vi "Round_Min_Max.vi"(8 "Binning 1":u32(ring)=4 items=["1"=1, "2"=2, "4"=4, "10"=10], 10 "CrsList":T1, 11 "Use Cursors":bool) -> (0 "min(Y)":u32, 1 "max(Y)":u32, 2 "min(X)":u32, 3 "max(X)":u32)   [LabVIEW 2013]
uses:
  <vilib>/Utility/miscctls.llb/LVCursorListTypeDef.ctl
panel:
  # "Binning"
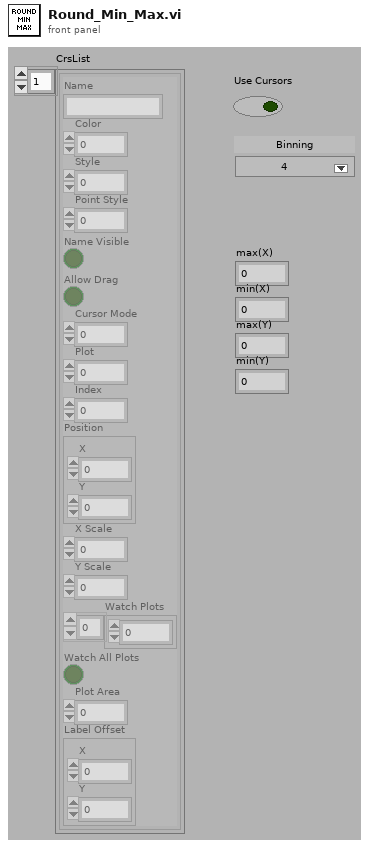
[diagram p1: front panel]
types:
  T1 = typedef "LVCursorListTypeDef.ctl" = cluster{"Name":string, "Color":u32, "Style":u8, "Point Style":u8, "Name Visible":bool, "Allow Drag":bool, "Cursor Mode":u32, "Plot":i32, "Index":i32, "Position":cluster{"X":dbl, "Y":dbl}, "X Scale":u32, "Y Scale":u32, "Watch Plots":i32[], "Watch All Plots":bool, "Plot Area":i32, "Label Offset":cluster{"X":dbl, "Y":dbl}}[]
  T2 = cluster{"Name":string, "Color":u32, "Style":u8, "Point Style":u8, "Name Visible":bool, "Allow Drag":bool, "Cursor Mode":u32, "Plot":i32, "Index":i32, "Position":cluster{"X":dbl, "Y":dbl}, "X Scale":u32, "Y Scale":u32, "Watch Plots":i32[], "Watch All Plots":bool, "Plot Area":i32, "Label Offset":cluster{"X":dbl, "Y":dbl}}
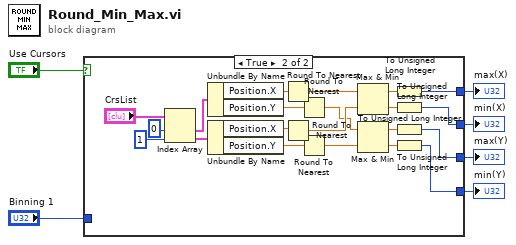
[diagram p0: block diagram]
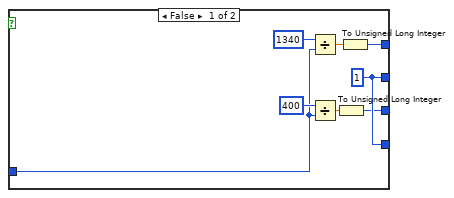
[diagram p2: hidden frame]
diagram:
  n1 = case shown="True" "Use Cursors" {
    tunnel: [w7 w18] -> w6
    tunnel: [w14 w15] -> w5
    tunnel: [w9 w16] -> w4
    tunnel: [w14 w17] -> w3
    tunnel: "Binning 1" -> [w11 _]
    frame False {
      w14 = u32 1
      n2 = Divide(x=u32 1340, y=w11) -> (x/y=w8:dbl)
      n3 = Divide(x=u32 400, y=w11) -> (x/y=w10:dbl)
      n4 = To Unsigned Long Integer(number=w10) -> (unsigned 32bit integer=w9:u32)
      n5 = To Unsigned Long Integer(number=w8) -> (unsigned 32bit integer=w7:u32)
    }
    frame True {
      n6 = Index Array(array="CrsList", index #1=0 ("index"), index #2=1 ("index")) -> (element #1=w21:T2, element #2=w22:T2)
      n7 = Unbundle By Name(w21) -> ("Position.X"=w23:dbl, "Position.Y"=w24:dbl)
      n8 = Unbundle By Name(w22) -> ("Position.X"=w25:dbl, "Position.Y"=w26:dbl)
      n9 = Round To Nearest(number=w23) -> (nearest integer value=w32:dbl)
      n10 = Round To Nearest(number=w25) -> (nearest integer value=w34:dbl)
      n11 = Round To Nearest(number=w24) -> (nearest integer value=w33:dbl)
      n12 = Round To Nearest(number=w26) -> (nearest integer value=w35:dbl)
      n13 = Max & Min(x=w32, y=w34) -> (max(x,y)=w28:dbl, min(x,y)=w29:dbl)
      n14 = Max & Min(x=w33, y=w35) -> (max(x,y)=w30:dbl, min(x,y)=w31:dbl)
      n15 = To Unsigned Long Integer(number=w28) -> (unsigned 32bit integer=w18:u32)
      n16 = To Unsigned Long Integer(number=w29) -> (unsigned 32bit integer=w17:u32)
      n17 = To Unsigned Long Integer(number=w30) -> (unsigned 32bit integer=w16:u32)
      n18 = To Unsigned Long Integer(number=w31) -> (unsigned 32bit integer=w15:u32)
    }
  }
  "max(X)" <- w6
  "min(X)" <- w3
  "max(Y)" <- w4
  "min(Y)" <- w5
